vi "Vision Processing.vi"(4 "error in (no error)":errorcluster, 7 "Image Size":T4=enum."320x240") -> ()   [LabVIEW 2015]
uses:
  Vision Support Code/Camera Types.ctl
  <vilib>/Rock Robotics/WPI/Camera/WPI_CameraImageSize.ctl
  <vilib>/Rock Robotics/WPI/Camera/WPI_CameraFrameRate.ctl
  <vilib>/Rock Robotics/WPI/Camera/WPI_CameraWhite Balance Values.ctl
  <vilib>/Rock Robotics/WPI/Camera/WPI_CameraExposure Values.ctl
  Robot Global Data.vi
  <vilib>/vision/NI_Vision_Development_Module.lvlib
panel:
  in  "Frame Rate (fps)":T1=30 min=1 max=30
  out "Highest Avg Score":dbl
  in  "Min Score Threshold":i32=75
  out "Detected Targets":T2(array[cluster]) {"Normalized Rect"."Numeric 5" format="%#_2g"; "Normalized Rect"."Numeric 3" format="%#_2g"; "Normalized Rect"."Numeric 2" format="%#_2g"; "Normalized Rect"."Numeric" format="%#_2g"}
  out "Sorted Particle Scores":T3(array[cluster]) {"Moment Factor" format="%#_3g"; "Aspect Ratio" format="%#_3g"; "Area to CH" format="%#_3g"; "X" format="%#_3g"; "Y" format="%#_3g"}
  in  "Display Original":bool=TRUE
  in  "Display Mask":bool=TRUE
  out "fps":dbl
  in  "Emphasize Limit Tests":bool=TRUE
  in  "Camera Type":T5=enum."MS HD3000 square"
  in  "Aspect Fudge Factor":dbl=1.0
  in  "Score Threshold":dbl=75.0
  out "ms to process":u32
  out "Qualified Particles":i32
  in  "LED Color":T6={"Hue"={23.67058792990901, 48.923317529462665}, "Sat"={66.78571428571429, 255.0}, "Val"={48.571428571428584, 255.0}} {"Hue" scale=0.0..255.0 scale format="%#_3g"}
  out "Masked":T7(plugin-control)
  out "Original Image":T7(plugin-control)
  # "This is only the initial camera size.\nOther camera setup is done\non the diagram. Notice it is set\nonce before the loop but can be\nupdated within the loop if needed."
  # "Instructions:\nUse LED Color to threshold and build particles. Adjust calibration if needed.\nDisplays are very useful for debugging, but will slow down execution, so you\nmay want to disable once working.\nAnnotations show the rectangle and the scores from top to bottom.\nChange camera setting on diagram."
  # "Density Profile"
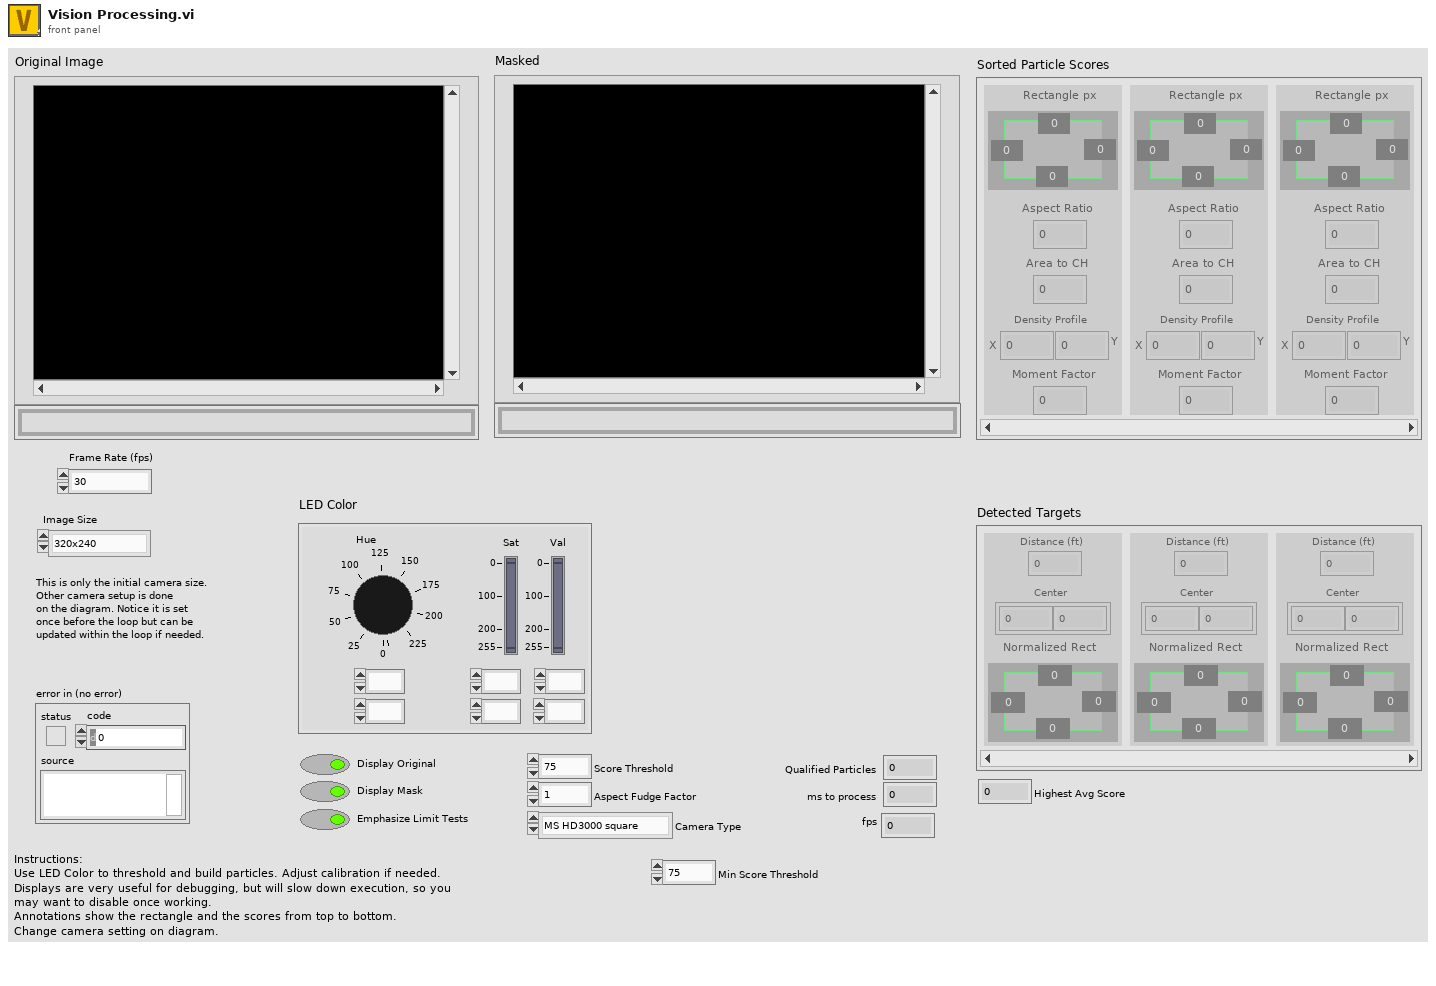
[diagram p1: front panel]
types:
  T1 = typedef "WPI_CameraFrameRate.ctl" = u32
  T2 = cluster{"Distance (ft)":dbl, "Center":cluster{dbl, dbl}, "Normalized Rect":cluster{"Numeric":dbl, "Numeric 2":dbl, "Numeric 3":dbl, "Numeric 5":dbl}}[]
  T3 = cluster{"Rectangle px":cluster{"Numeric":dbl, "Numeric 2":dbl, "Numeric 3":dbl, "Numeric 5":dbl}, "Aspect Ratio":dbl, "Area to CH":dbl, "X":dbl, "Y":dbl, "Moment Factor":dbl}[]
  T4 = typedef "WPI_CameraImageSize.ctl" = enum16{"640x480", "320x240", "160x120", "Custom"}
  T5 = typedef "Camera Types.ctl" = enum16{"206", "1011", "1013", "MS HD3000 square", "MS HD3000 640x480"}
  T6 = cluster{"Hue":cluster{dbl, dbl}, "Sat":cluster{dbl, dbl}, "Val":cluster{dbl, dbl}}
  T7 = typedef "IMAQ Image.ctl" = refnum<image>
  T8 = typedef "WPI_CameraExposure Values.ctl" = enum16{"Auto", "Flicker-free 50 Hz", "Flicker-free 60 Hz", "Hold current", "Custom"}
  T9 = typedef "WPI_CameraWhite Balance Values.ctl" = enum16{"Auto", "Fixed indoor", "Fixed outdoor 1", "Fixed outdoor 2", "Fixed fluorescent 1", "Fixed fluorescent 2", "Hold current", "Custom"}
  T10 = typedef "Particle Parameters" = i32
  T11 = typedef "Image Type" = u32
  T12 = typedef "WPI_CameraDevRef.ctl" = cluster{"Camera Address":string, "CameraStatus":errorcluster}
  T13 = cluster{"Bounding box":cluster{"left":dbl, "top":dbl, "right":dbl, "bottom":dbl}, "Aspect Ratio":dbl, "Area to CH":dbl, "X Mask":dbl, "Y Mask":dbl, "Moment":dbl}[]
  T14 = cluster{"Rectangle":cluster{"Numeric":dbl, "Numeric 2":dbl, "Numeric 3":dbl, "Numeric 5":dbl}, "L":dbl, "Area to CH":dbl, "X":dbl, "Y":dbl, "Moment Factor":dbl}[]
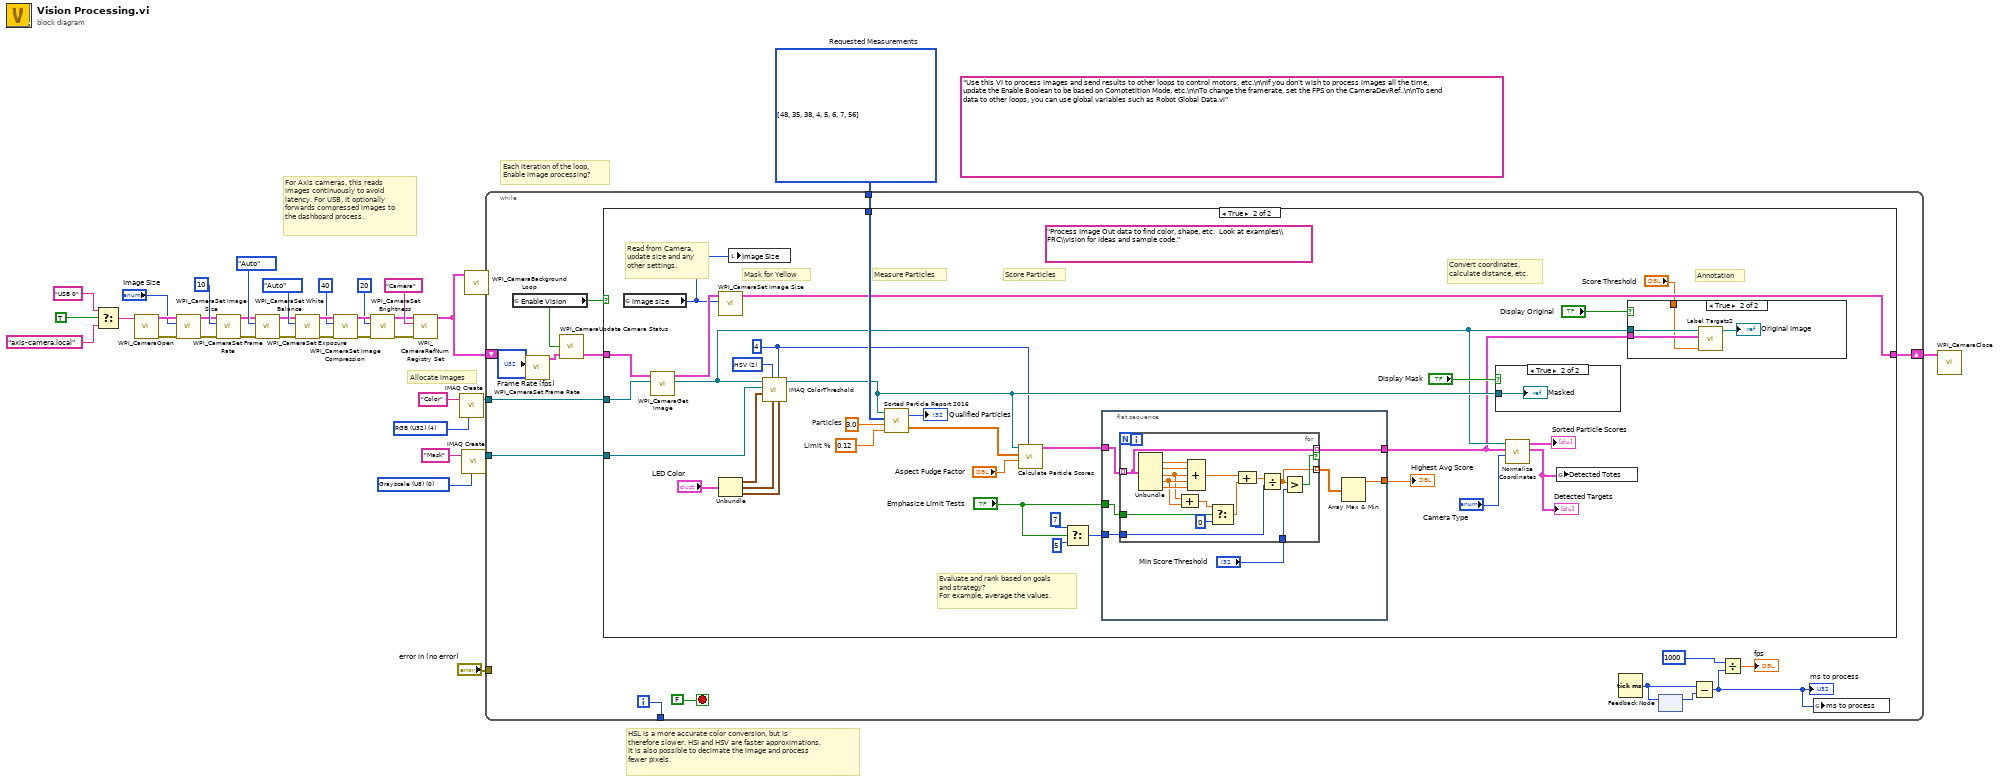
[diagram p0: block diagram]
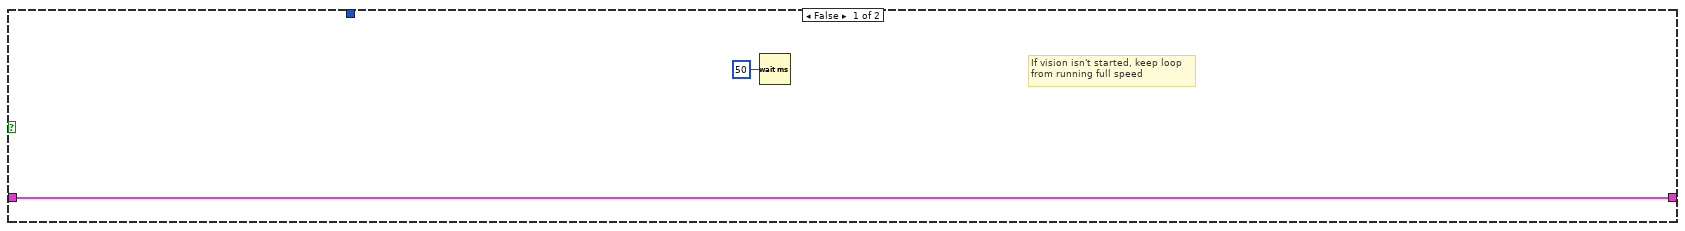
[diagram p2: hidden frame]
diagram:
  (unwired) "Use this VI to process images and send results to other loops to control motors, etc.\n\nIf you don't wish to process images all the time, update the Enable Boolean to be based on Comptetition Mode, etc.\n\nTo change the framerate, set the FPS on the CameraDevRef..\n\nTo send data to other loops, you can use global variables such as Robot Global Data.vi"
  w29 = T10[] [48, 35, 38, 4, 5, 6, 7, 56] items=["Center of Mass X", "Center of Mass Y", "First Pixel X", "First Pixel Y", "Bounding Rect Left", "Bounding Rect Top", "Bounding Rect Right", "Bounding Rect Bottom", "Max Feret Diameter Start X", "Max Feret Diameter Start Y", "Max Feret Diameter End X", "Max Feret Diameter End Y", "Max Horiz. Segment Length Left", "Max Horiz. Segment Length Right", "Max Horiz. Segment Length Row", "-", "Bounding Rect Width", "Bounding Rect Height", "Bounding Rect Diagonal", "Perimeter", "Convex Hull Perimeter", "Holes' Perimeter", "Max Feret Diameter", "Equivalent Ellipse Major Axis", "Equivalent Ellipse Minor Axis", "Equivalent Ellipse Minor Axis (Feret)", "Equivalent Rect Long Side", "Equivalent Rect Short Side", "Equivalent Rect Diagonal", "Equivalent Rect Short Side (Feret)", "Average Horiz. Segment Length", "Average Vert. Segment Length", "Hydraulic Radius", "Waddel Disk Diameter", "-", "Area", "Holes' Area", "Particle & Holes' Area", "Convex Hull Area", "Image Area", "-", "Number of Holes", "Number of Horiz. Segments", "Number of Vert. Segments", "-", "Orientation", "Max Feret Diameter Orientation", "-", "% Area/Image Area", "% Area/(Particle & Holes' Area)", "Ratio of Equivalent Ellipse Axes", "Ratio of Equivalent Rect Sides", "-", "Elongation Factor", "Compactness Factor", "Heywood Circularity Factor", "Type Factor", "-", "Sum X", "Sum Y", "Sum XX", "Sum XY", "Sum YY", "Sum XXX", "Sum XXY", "Sum XYY", "Sum YYY", "-", "Moment of Inertia XX", "Moment of Inertia XY", "Moment of Inertia YY", "Moment of Inertia XXX", "Moment of Inertia XXY", "Moment of Inertia XYY", "Moment of Inertia YYY", "Norm. Moment of Inertia XX", "Norm. Moment of Inertia XY", "Norm. Moment of Inertia YY", "Norm. Moment of Inertia XXX", "Norm. Moment of Inertia XXY", "Norm. Moment of Inertia XYY", "Norm. Moment of Inertia YYY", "Hu Moment 1", "Hu Moment 2", "Hu Moment 3", "Hu Moment 4", "Hu Moment 5", "Hu Moment 6", "Hu Moment 7"]  # Requested Measurements
  w32 = T11 0 items=["Grayscale (U8)", "Grayscale (I16)", "Grayscale (SGL)", "Complex (CSG)", "RGB (U32)", "HSL (U32)", "RGB (U64)", "Grayscale (U16)"] ("Image Type")
  w34 = T11 4 items=["Grayscale (U8)", "Grayscale (I16)", "Grayscale (SGL)", "Complex (CSG)", "RGB (U32)", "HSL (U32)", "RGB (U64)", "Grayscale (U16)"] ("Image Type")
  # "Each iteration of the loop,\nEnable image processing?"
  # "HSL is a more accurate color conversion, but is\ntherefore slower. HSI and HSV are faster approximations.\nIt is also possible to decimate the image and process\nfewer pixels."
  # "For Axis cameras, this reads\nimages continuously to avoid\nlatency. For USB, it optionally\nforwards compressed images to\nthe dashboard process."
  # "Allocate images"
  n1 = Select(t="USB 0" ("format string"), s=TRUE ("dot notation? (F)"), f="axis-camera.local" ("format string")) -> (s? t:f=w28:string)
  n2 = call <vilib>:"WPI_CameraOpen.vi"("Camera Address"=w28) -> ("error out"=w16:errorcluster, "CameraDevRef"=w15:T12)  [unwired: 1 in, 8 out]
  n3 = call <vilib>:"WPI_CameraSet Image Size.vi"("error in (no error)"=w16, "Image Size"="Image Size", "CameraDevRef"=w15) -> ("error out"=w17:errorcluster, "CameraDevRef Out"=w14:T12)  [unwired: 1 in, 6 out]
  n4 = call <vilib>:"WPI_CameraSet Frame Rate.vi"("error in (no error)"=w17, "Frame Rate (fps)"=T1 10, "CameraDevRef"=w14) -> ("error out"=w18:errorcluster, "CameraDevRef Out"=w12:T12)  [unwired: 7 out]
  n5 = call <vilib>:"WPI_CameraSet White Balance.vi"("error in (no error)"=w18, "White Balance"=WPI_CameraWhite_Balance_Values."Auto", "CameraDevRef"=w12) -> ("error out"=w19:errorcluster, "CameraDevRef Out"=w13:T12)  [unwired: 1 in, 6 out]
  n6 = call <vilib>:"WPI_CameraSet Exposure.vi"("error in (no error)"=w19, "Exposure"=WPI_CameraExposure_Values."Auto", "CameraDevRef"=w13) -> ("error out"=w20:errorcluster, "CameraDevRef Out"=w10:T12)  [unwired: 1 in, 6 out]
  n7 = call <vilib>:"WPI_CameraSet Image Compression.vi"("error in (no error)"=w20, "Compression"=40, "CameraDevRef"=w10) -> ("error out"=w21:errorcluster, "CameraDevRef Out"=w11:T12)  [unwired: 7 out]
  n8 = call <vilib>:"WPI_CameraSet Brightness.vi"("error in (no error)"=w21, "Brightness"=20, "CameraDevRef"=w11) -> ("error out"=w22:errorcluster, "CameraDevRef Out"=w1:T12)  [unwired: 7 out]
  n9 = call <vilib>:"WPI_CameraRefNum Registry Set.vi"("error in (no error)"=w22, "refnum name"="Camera", "CameraDevRef"=w1) -> ("CameraDevRef"=w6:T12)  [unwired: 1 in, 7 out]
  n10 = call "IMAQ Create"("Image Name"="Color", "Image Type"=w34) -> ("New Image"=w33:T7)  [unwired: 2 in, 2 out]
  n11 = call "IMAQ Create"("Image Name"="Mask", "Image Type"=w32) -> ("New Image"=w30:T7)  [unwired: 2 in, 2 out]
  n12 = call <vilib>:"WPI_CameraBackground Loop.vi"("CameraDevRef"=w6) -> ()  [unwired: 11 in]
  n13 = while {
    tunnel: w33 -> [w46]
    tunnel: w30 -> [w50]
    tunnel: w29 -> [w49]
    tunnel: "error in (no error)" -> [_]
    tunnel: [w45] -> _
    shift-right: [w42] -> w2
    shift-left: w6 -> [w37]
    i -> [w45]
    stop <- FALSE stop-if-true
    n14 = global read "Robot Global Data.vi" "Enable Vision"() -> (w44:bool)
    n15 = call <vilib>:"WPI_CameraSet Frame Rate.vi"("Frame Rate (fps)"="Frame Rate (fps)", "CameraDevRef"=w37) -> ("CameraDevRef Out"=w38:T12)  [unwired: 1 in, 8 out]
    n16 = call <vilib>:"WPI_CameraUpdate Camera Status.vi"("CameraDevRef In"=w38, "Enable Vision"=w44) -> ("CameraDevRef Out"=w43:T12)  [unwired: 3 in]
    n17 = case shown="True" w44 {
      tunnel: w50 -> [_ w86]
      tunnel: w49 -> [_ w81]
      tunnel: w43 -> [w52 w77]
      tunnel: w46 -> [_ w76]
      tunnel: [w52 w74] -> w42
      frame False {
        # "If vision isn't started, keep loop\nfrom running full speed"
        n18 = Wait (ms)(milliseconds to wait=u32 50) -> ()  [unwired: 1 out]
      }
      frame True {
        w57 = 4 ("Replace Value")
        w71 = u16 2 items=["RGB", "HSL", "HSV", "HSI"] ("Color Mode")
        (unwired) "Process Image Out data to find color, shape, etc.  Look at examples\\FRC\\vision for ideas and sample code."
        w78 = 0.12  # Limit %
        w80 = 3.0  # Particles
        # "Evaluate and rank based on goals\nand strategy?\nFor example, average the values."
        # "Read from Camera,\nupdate size and any\nother settings."
        # "Measure Particles"
        # "Convert coordinates,\ncalculate distance, etc."
        # "Annotation"
        # "Score Particles"
        # "Mask for Yellow"
        n19 = global read "Robot Global Data.vi" "image size"() -> (w55:T4)
        n20 = call <vilib>:"WPI_CameraGet Image.vi"("Image"=w76, "CameraDevRef"=w77) -> ("Image Out"=w60:T7, "CameraDevRef Out"=w75:T12)  [unwired: 7 in, 1 out]
        n21 = call <vilib>:"WPI_CameraSet Image Size.vi"("Image Size"=w55, "CameraDevRef"=w75) -> ("CameraDevRef Out"=w74:T12)  [unwired: 2 in, 7 out]
        n22 = Unbundle("LED Color") -> ("Hue"=w85:cluster{dbl, dbl}, "Sat"=w84:cluster{dbl, dbl}, "Val"=w83:cluster{dbl, dbl})
        n23 = local write "Image Size"(w55) -> ()
        n24 = call "IMAQ ColorThreshold"("Blue or Luma or Val or Inten Range"=w83, "Replace Value"=w57, "Green or Sat Range"=w84, "Color Mode"=w71, "Red or Hue Range"=w85, "Image Dst"=w86, "Image Src"=w60) -> ("Image Dst Out"=w70:T7)  [unwired: 3 in, 1 out]
        n25 = call "Sorted Particle Report 2016.vi"("Min Area Size %"=w78, "Particle Count Limit"=w80, "Pixel Measurements"=w81, "Image in"=w70) -> ("Sorted Data"=w69:dbl[][], "Particles"=→"Qualified Particles":i32)
        n26 = call "Calculate Particle Scores.vi"("Pixel Value"=w57, "Aspect Fudge Factor"="Aspect Fudge Factor", "Sorted Data"=w69, "Image in"=w70) -> ("Scores"=w67:T13)  [unwired: 7 in]
        n27 = Select(t=7, s="Emphasize Limit Tests", f=5) -> (s? t:f=w64:i32)
        n28 = flat-sequence {
          tunnel: w67 -> [w97]
          tunnel: w64 -> [w95]
          tunnel: [w98] -> w63
          tunnel: [w92] -> w59
          tunnel: "Emphasize Limit Tests" -> [w96]
          frame #0 {
            n29 = for {
              tunnel: w97 -> [w112] mode=indexing
              tunnel: [w112] -> w92 mode=indexing if=w111
              tunnel: [w110] -> w93 mode=indexing
              tunnel: w95 -> [w109]
              tunnel: "Min Score Threshold" -> [w108]
              tunnel: w96 -> [w101]
              n30 = Unbundle(w112) -> ("Aspect Ratio"=w114:dbl, "Area to CH"=w113:dbl, "X Mask"=w103:dbl, "Y Mask"=w104:dbl, "Moment"=w105:dbl)  [unwired: 1 out]
              n31 = Compound Arithmetic op=ADD(w103, w104) -> (w102:dbl)
              n32 = Compound Arithmetic op=ADD(w114, w113, w103, w104, w105) -> (w107:dbl)
              n33 = Select(t=w102, s=w101, f=0) -> (s? t:f=w100:dbl)
              n34 = Compound Arithmetic op=ADD(w107, w100) -> (w106:dbl)
              n35 = Divide(x=w106, y=w109) -> (x/y=w110:dbl)
              n36 = Greater?(x=w110, y=w108) -> (0:w111:bool)
            }
            n37 = Array Max & Min(array=w93) -> (max value=w98:dbl)  [unwired: 3 out]
          }
        }
        n38 = case shown="True" "Display Mask" {
          tunnel: w70 -> [_ w91]
          frame False {
          }
          frame True {
            "Masked" <- w91
          }
        }
        n39 = call "Normalize Coordinates.vi"("Camera Type"="Camera Type", "Targets"=w59, "Image in"=w60) -> ("Found Targets"=w56:T2, "Sorted Scores"=→"Sorted Particle Scores":T14)  [unwired: 7 in]
        "Detected Targets" <- w56
        n40 = global write "Robot Global Data.vi" "Detected Totes"(w56) -> ()
        n41 = case shown="True" "Display Original" {
          tunnel: w60 -> [_ w90]
          tunnel: w59 -> [_ w88]
          tunnel: "Score Threshold" -> [_ w87]
          frame False {
          }
          frame True {
            n42 = call "Label Targets2.vi"("Score Threshold"=w87, "Targets"=w88, "Image in"=w90) -> ("Image out"=→"Original Image":T7)  [unwired: 8 in]
          }
        }
        "Highest Avg Score" <- w63
      }
    }
    n43 = Tick Count (ms)() -> (millisecond timer value=w47:u32)
    n44 = feedback-in #1(w47) -> ()
    n45 = feedback #1() -> (w48:u32)  [unwired: 1 in]
    n46 = Subtract(x=w47, y=w48) -> (x-y=w41:u32)
    "ms to process" <- w41
    n47 = Divide(x=1000 ("Brightness"), y=w41) -> (x/y=→"fps":dbl)
    n48 = global write "Robot Global Data.vi" "ms to process"(w41) -> ()
  }
  n49 = call <vilib>:"WPI_CameraClose.vi"("CameraDevRef"=w2) -> ()  [unwired: 1 in, 10 out]
